vi "Pre Launch Init.vi"(11 "Debug UI in":refnum<class "Debug UI.lvclass">) -> (0 "error out":errorcluster, 3 "Debug UI out":refnum<class "Debug UI.lvclass">)   [LabVIEW 2016, in "Assert API Components.lvlib" / "Log Assert Core.lvlib" / "Debug UI.lvclass"]
doc: "(<B>Filename</B>: Actor Framework.lvlib:Actor.lvclass:Pre Launch Init.vi)\n\nDefines behavior that occurs after the Launch Nested Actor method is invoked but before the actor's Actor Core method begins running.\n\nBy default, this method does nothing. A descendant class may override it to define behavior."
uses:
  Debug UI.lvclass
  Debug UI.lvclass/Debug UI.ctl
  LAC Error Logger/LAC Error Logger.lvclass
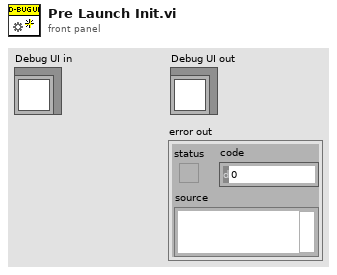
[diagram p1: front panel]
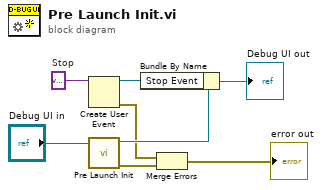
[diagram p0: block diagram]
diagram:
  w6 = variant  # Stop
  n1 = Create User Event(user event datatype=w6) -> (user event=w4:refnum<user-event>, error out=w2:errorcluster)  [unwired: 1 in]
  n2 = call-parent "Pre Launch Init.vi"("Actor in"="Debug UI in") -> ("error out"=w8:errorcluster, "Actor out"=w7:refnum<class "Debug UI.lvclass">)  [unwired: 9 in]
  n3 = Bundle By Name(cluster=w7, "Stop Event"=w4) -> (→"Debug UI out":refnum<class "Debug UI.lvclass">)
  n4 = Merge Errors(w2, w8) -> (→"error out":errorcluster)
